vi "camara.vi"() -> ()   [LabVIEW 2010]
uses:
  <vilib>/addons/PixeLINK/Low Level Functions/CAMERA_FEATURES.llb/TDPU-CameraFeatures-PixelFormat.ctl
  <vilib>/vision/Image Controls.llb/IMAQ Image.ctl
panel:
  in  "Nueva Linea?":bool
  out "Contraste2":dbl
  out "Line Profile":dbl[](graph)
  out "Gray Level Intensities":T1 {"Standard  Deviation" format="%.2f"; "Mean Intensity" format="%.2f"; "Maximum Intensity" format="%.2f"; "Minimum Intensity" format="%.2f"}
  out "time(ms)":u32
  in  "Tab Control":enum32{"Camara"}(tab)
  in  "Selector":u16(ring) items=["776002034"]
  in  "Streeam?":bool
  out "Camara Funciona?":bool
  out "Contraste":dbl(graph)
  out "Image":T2(plugin-control)
  in  "Grabar":bool
  in  "Camera Parameters":T4 {"Pixel Format" items=["PIXEL_FORMAT_MONO8", "PIXEL_FORMAT_MONO16", "PIXEL_FORMAT_YUV422", "PIXEL_FORMAT_BAYER8_GRBG", "PIXEL_FORMAT_BAYER16_GRBG", "PIXEL_FORMAT_RGB24", "PIXEL_FORMAT_RGB48", "PIXEL_FORMAT_BAYER8_RGGB", "PIXEL_FORMAT_BAYER8_GBRG ", "PIXEL_FORMAT_BAYER8_BGGR ", "PIXEL_FORMAT_BAYER16_RGGB ", "PIXEL_FORMAT_BAYER16_GBRG", "PIXEL_FORMAT_BAYER16_BGGR", "PIXEL_FORMAT_RGB32"]}
  in  "stop":bool
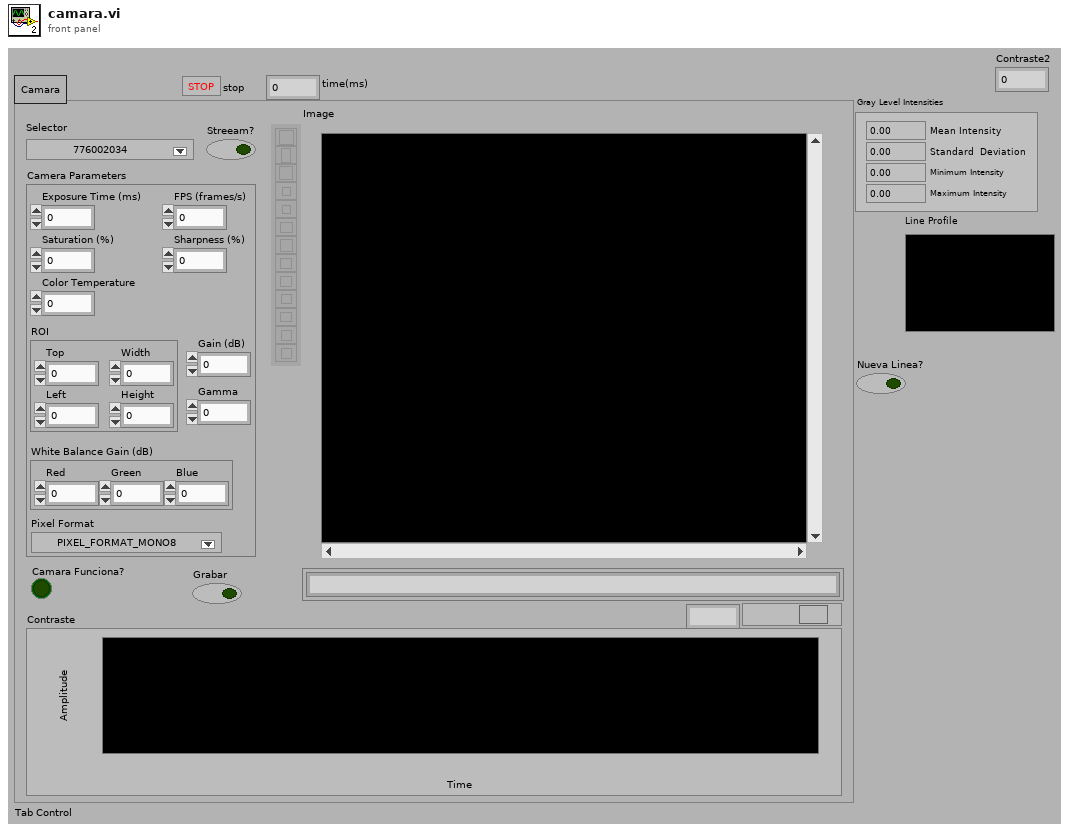
[diagram p1: front panel]
types:
  T1 = cluster{"Mean Intensity":sgl, "Standard  Deviation":sgl, "Minimum Intensity":sgl, "Maximum Intensity":sgl}
  T2 = typedef "IMAQ Image.ctl" = refnum<image>
  T3 = typedef "TDPU-CameraFeatures-PixelFormat.ctl" = u16
  T4 = cluster{"Exposure Time (ms)":dbl, "Gain (dB)":dbl, "Saturation (%)":dbl, "Sharpness (%)":dbl, "Color Temperature":dbl, "ROI":cluster{"Top":i32, "Left":i32, "Width":i32, "Height":i32}, "White Balance Gain (dB)":cluster{"Red":dbl, "Green":dbl, "Blue":dbl}, "Gamma":dbl, "Pixel Format":T3, "FPS (frames/s)":i32}
  T5 = cluster{"hCamera":u32, "Error":errorcluster, "uSerialNumber OUT":u32}
  T6 = cluster{"hCamera":u32, "Error":errorcluster, "uSerialNumber":u32}
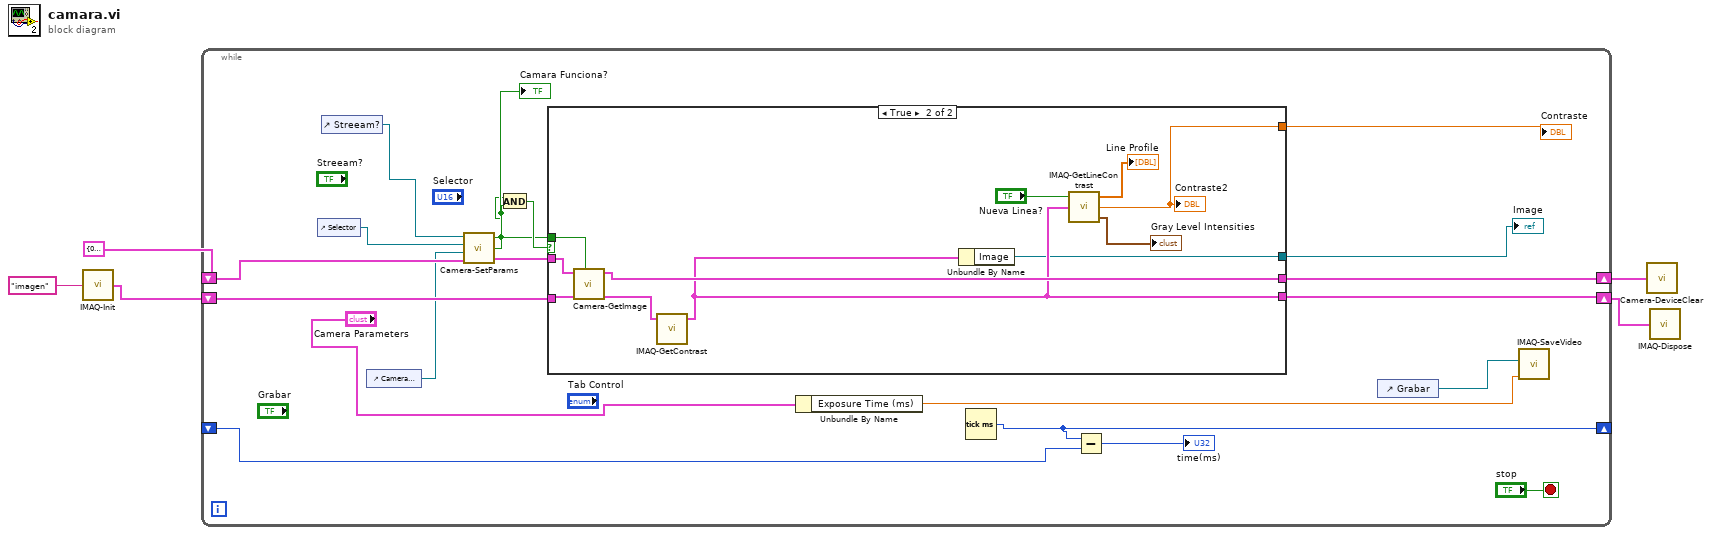
[diagram p0: block diagram]
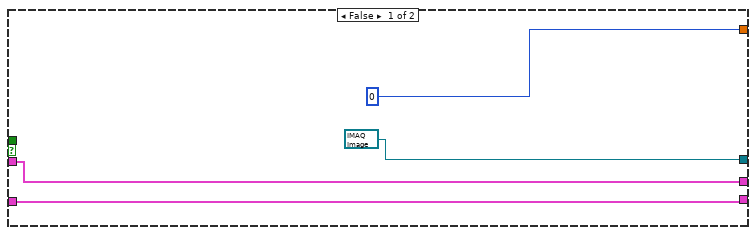
[diagram p2: hidden frame]
diagram:
  n1 = call "IMAQ-Init.vi"("Image Name"="imagen") -> ("Image Device IN"=w4:cluster{"Image":T2, "errorImage":errorcluster})
  n2 = while {
    shift-right: [w18] -> w1
    shift-left: w4 -> [w21]
    shift-right: [w20] -> w2
    shift-left: T5 {"hCamera"=0, "Error"={"status"=FALSE, "code"=0, "source"=""}, "uSerialNumber OUT"=0} ("Camera Device  IN") -> [w19]
    shift-right: [w12] -> _
    shift-left: _ -> [w11]
    stop <- "stop" stop-if-true
    n3 = control-ref of="Selector"() -> (w24:refnum<vi>)
    n4 = control-ref of="Streeam?"() -> (w23:refnum<vi>)
    n5 = control-ref of="Camera Parameters"() -> (w7:refnum<vi>)
    n6 = call "Camera-SetParams.vi"("Camera Device  IN"=w19, "Camera Parameters"=w7, "Selector"=w24, "Stream?"=w23) -> ("Camera Device OUT"=w22:T6, "Funciona?"=w16:bool, "Stream? OUT"=w15:bool)
    "Camara Funciona?" <- w16
    n7 = And(x=w15, y=w16) -> (x .and. y?=w17:bool)
    n8 = case shown="True" w17 {
      tunnel: w22 -> [w29 w39]
      tunnel: w15 -> [_ w40]
      tunnel: w21 -> [w28 w38]
      tunnel: [w29 w37] -> w20
      tunnel: [w28 w32] -> w18
      tunnel: [u32 0 ("Numeric") w30] -> w14
      tunnel: [T2 refnum ("Image") w31] -> w6
      frame False {
      }
      frame True {
        n9 = call "Camera-GetImage.vi"("Streeam"=w40, "Image Device IN"=w38, "Camera Device IN"=w39) -> ("Image Device OUT"=w36:cluster{"Image":T2, "errorImage":errorcluster}, "Camera Device OUT"=w37:T6)  [unwired: 4 in]
        n10 = call "IMAQ-GetContrast.vi"("Image Device IN"=w36) -> ("Image Device OUT"=w32:cluster{"Image":T2, "errorImage":errorcluster})  [unwired: 3 in, 1 out]
        n11 = Unbundle By Name(w32) -> ("Image"=w31:T2)
        n12 = call "IMAQ-GetLineContrast.vi"("Image Device"=w32, "Nueva Linea?"="Nueva Linea?") -> ("Gray Level Intensities"=→"Gray Level Intensities":T1, "Contraste"=w30:dbl, "Line Profile"=→"Line Profile":dbl[])  [unwired: 1 in]
        "Contraste2" <- w30
      }
    }
    "Image" <- w6
    "Contraste" <- w14
    n13 = Unbundle By Name("Camera Parameters") -> ("Exposure Time (ms)"=w13:dbl)
    n14 = Tick Count (ms)() -> (millisecond timer value=w12:u32)
    n15 = Subtract(x=w12, y=w11) -> (x-y=→"time(ms)":u32)
    n16 = control-ref of="Grabar"() -> (w9:refnum<vi>)
    n17 = call "IMAQ-SaveVideo.vi"("Exposure Time (ms)"=w13, "Grabar"=w9) -> ()  [unwired: 2 in, 1 out]
  }
  n18 = call "Camera-DeviceClear.vi"("Camera Device OUT"=w2) -> ()
  n19 = call "IMAQ-Dispose.vi"("Image Device IN"=w1) -> ()
